vi "Receiver HMI Main.vi"() -> ()   [LabVIEW 2025]
uses:
  <vilib>/Instr/_visa.llb/VISA Configure Serial Port (Instr).vi
  <vilib>/picture/picture.llb/Draw True-Color Pixmap.vi
panel:
  out "Barcode":bool
  out "unsigned byte array":u8[](array[numeric])
  out "Wire":bool
  out "Motor":bool
  out "Light":bool
  out "Touch":bool
  out "Solenoid":bool
  out "Cancelled":bool
  out "Receive Buffer":string
  in  "Enable Wire":bool
  in  "Enable Barcode":bool
  in  "Enable Motor":bool
  in  "Enable Light":bool
  in  "Enable Touch":bool
  in  "Enable Solenoid":bool
  out "String":string
  out "2D Picture":picture
  out "Receiving Progress:":dbl(slide) scale=0.0..100.0
  # "RECEIVER"
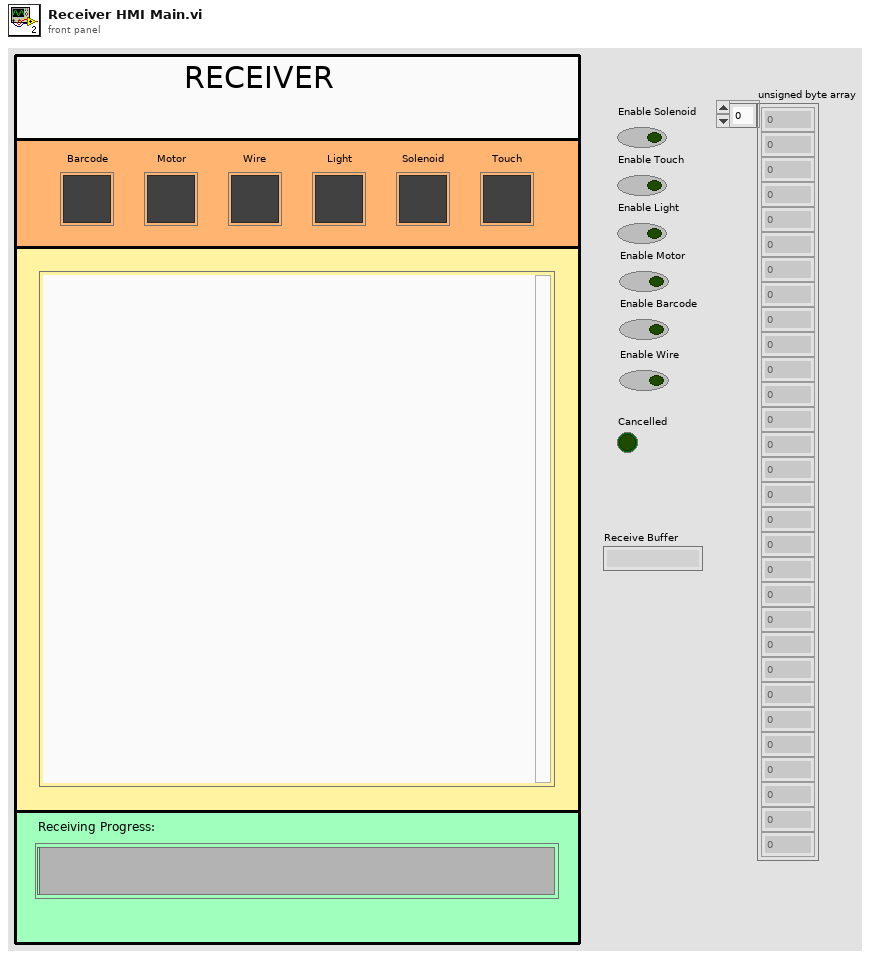
[diagram p1: front panel]
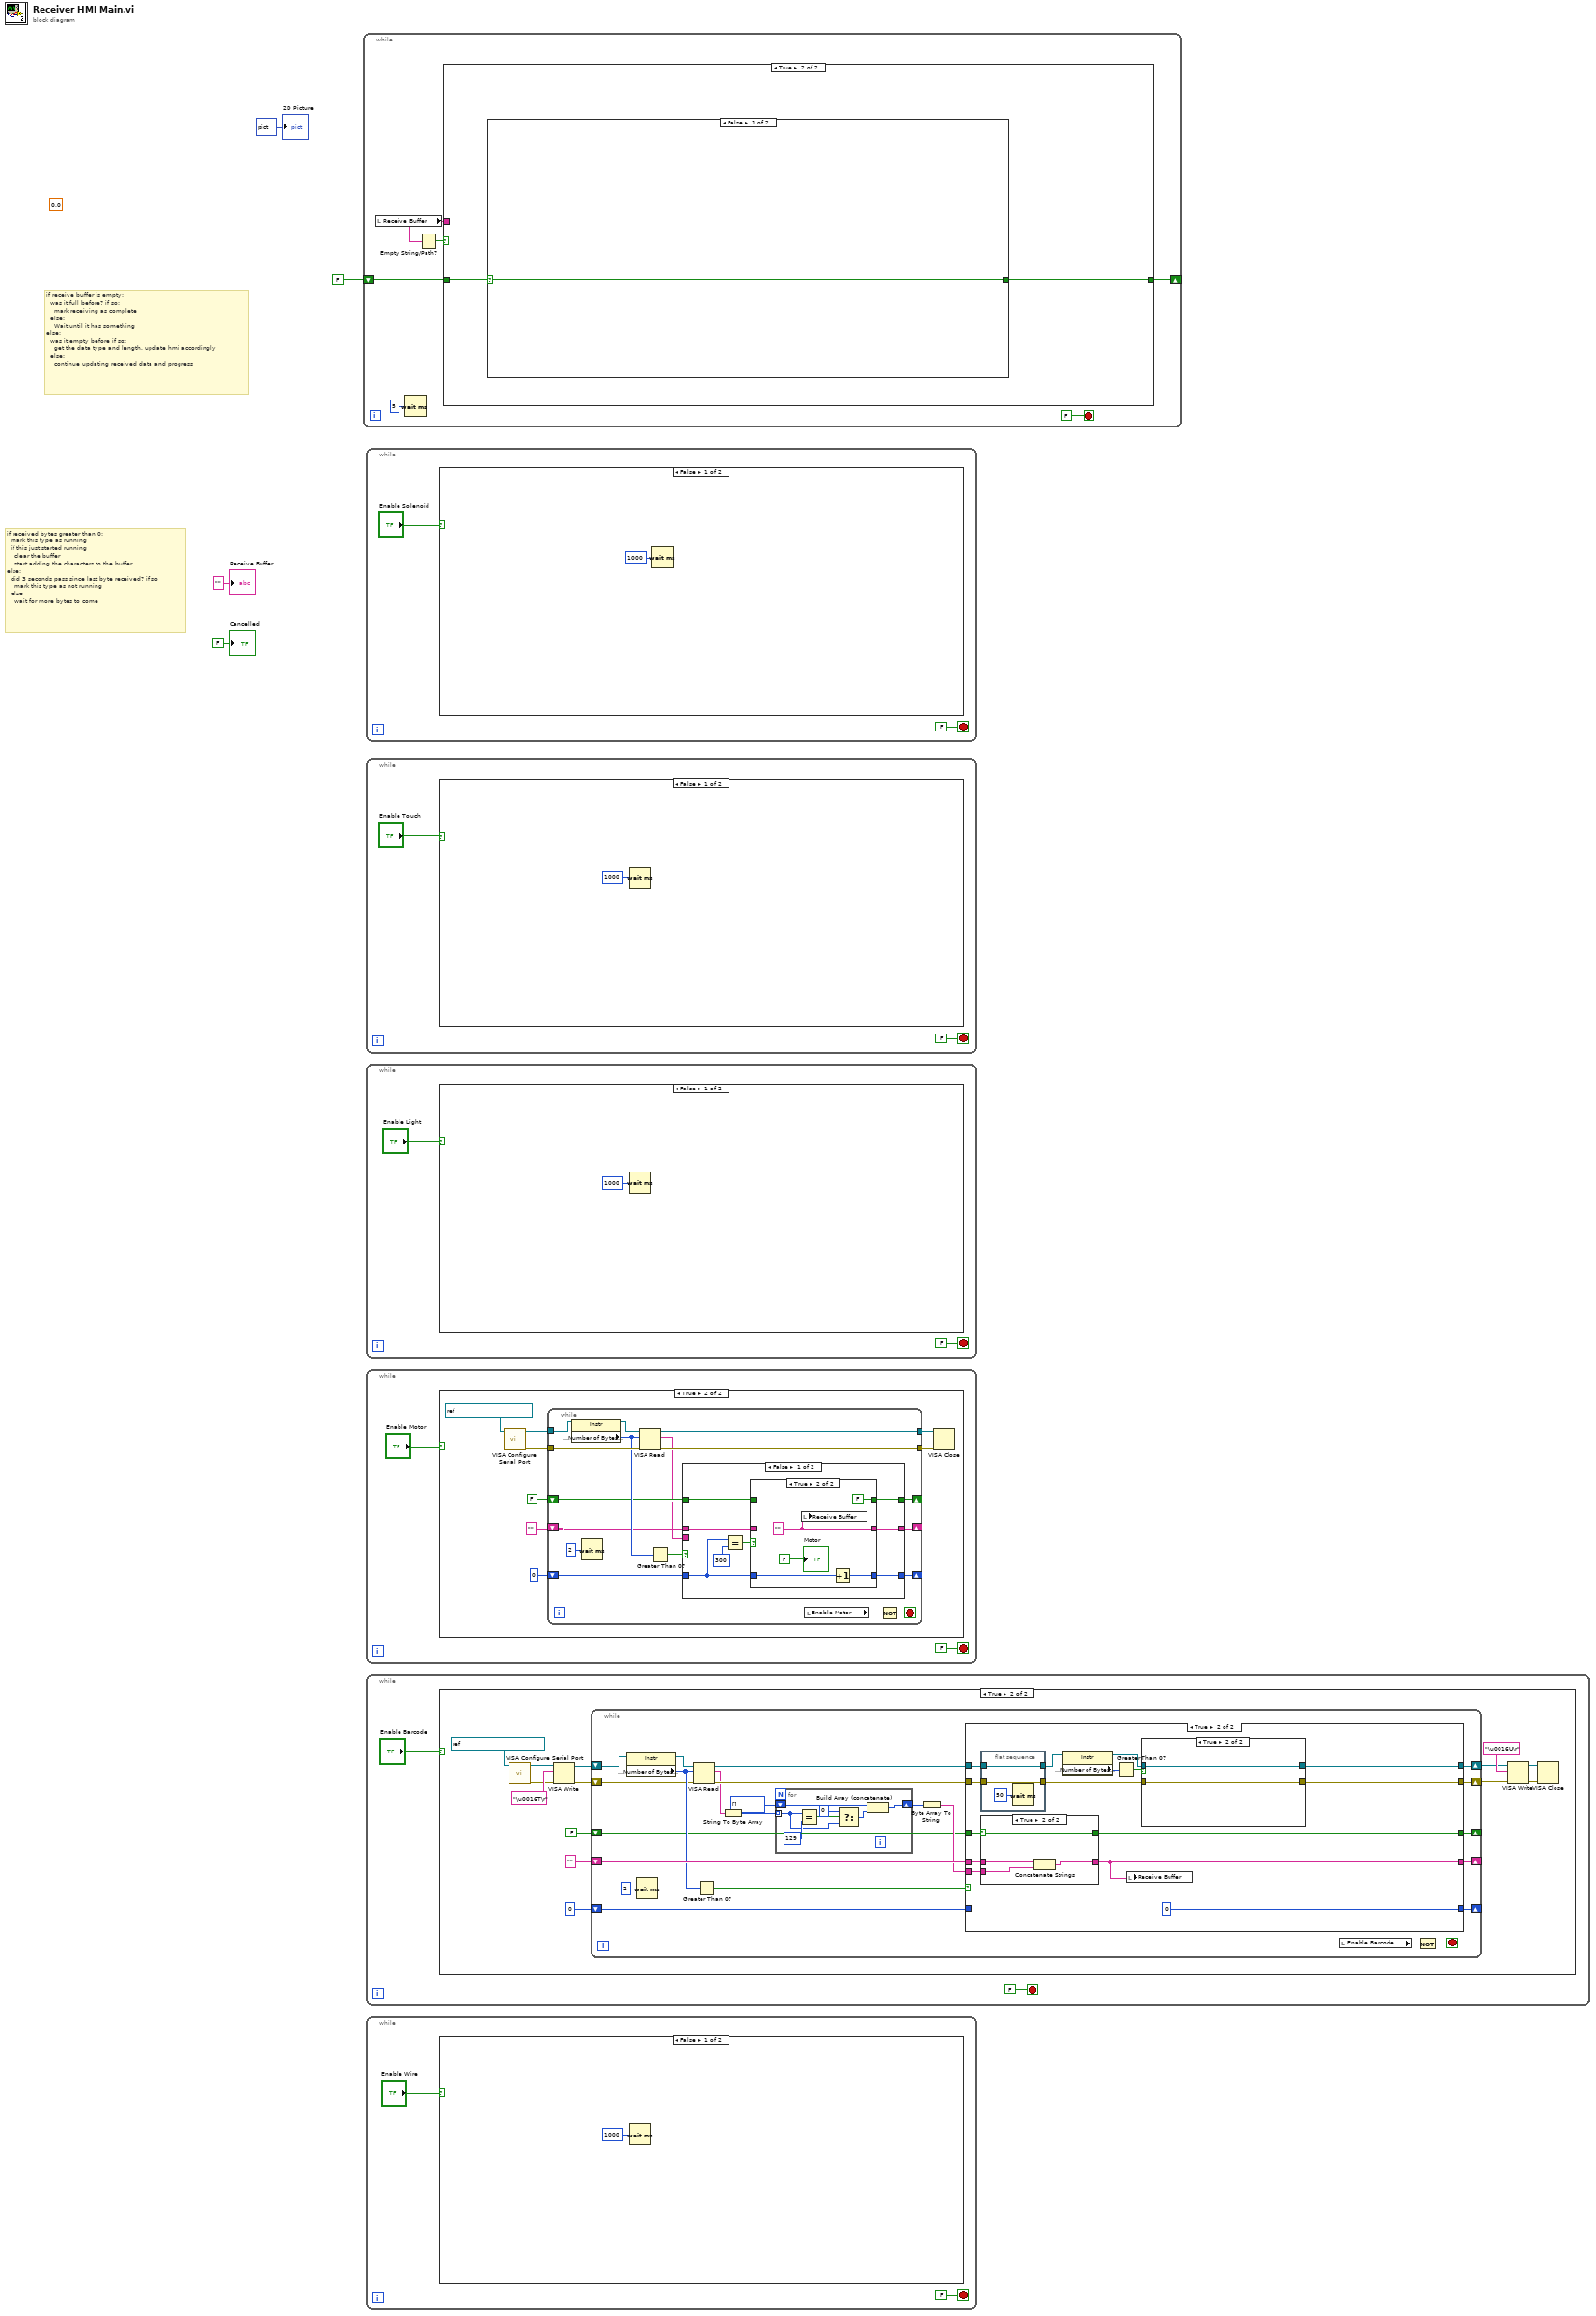
[diagram p0: block diagram]
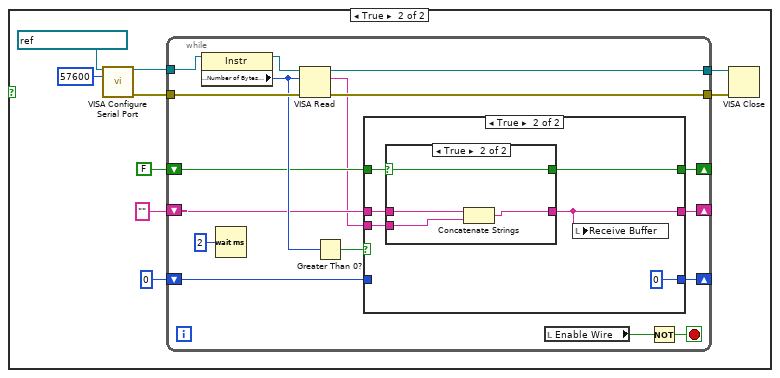
[diagram p2: hidden frame]
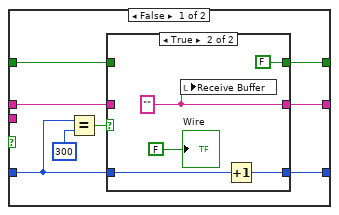
[diagram p3: hidden frame]
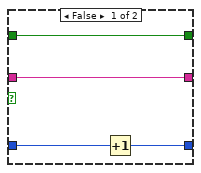
[diagram p4: hidden frame]
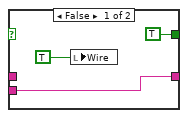
[diagram p5: hidden frame]
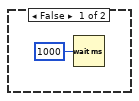
[diagram p6: hidden frame]
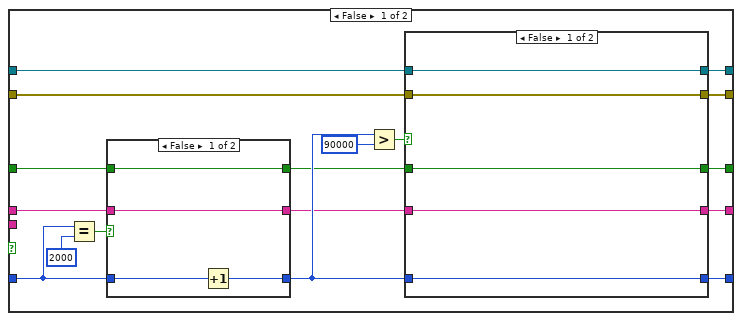
[diagram p7: hidden frame]
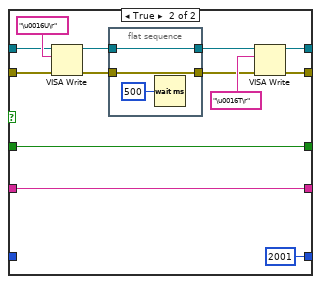
[diagram p8: hidden frame]
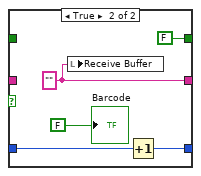
[diagram p9: hidden frame]
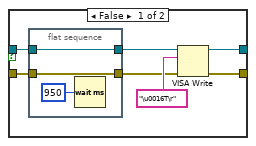
[diagram p10: hidden frame]
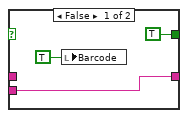
[diagram p11: hidden frame]
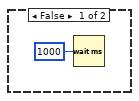
[diagram p12: hidden frame]
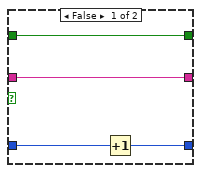
[diagram p13: hidden frame]
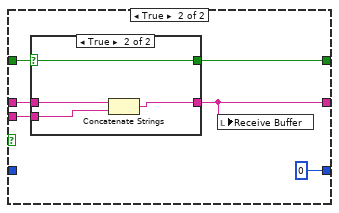
[diagram p14: hidden frame]
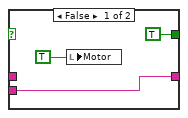
[diagram p15: hidden frame]
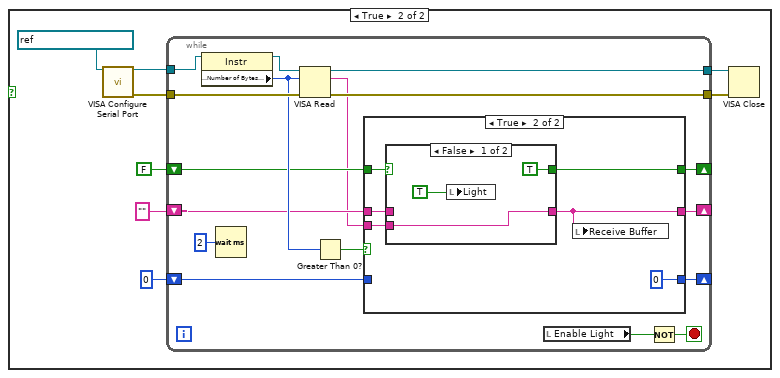
[diagram p16: hidden frame]
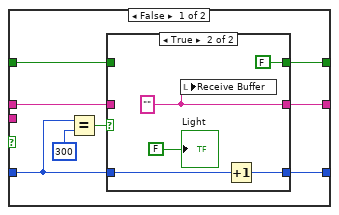
[diagram p17: hidden frame]
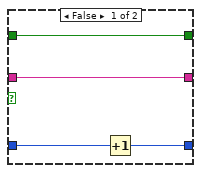
[diagram p18: hidden frame]
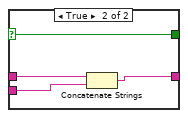
[diagram p19: hidden frame]
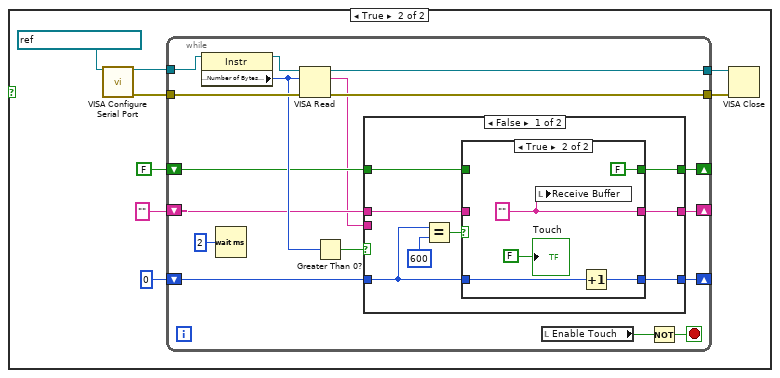
[diagram p20: hidden frame]
diagram:
  (unwired) 0.0 ("Receiving Progress:")
  # "if receive buffer is empty:\n  was it full before? if so:\n    mark receiving as complete\n  else:\n    Wait until it has something\nelse:\n  was it empty before if so:\n    get the data type and length. update hmi accordingly\n  else:\n    continue updating received data and progress"
  # "if received bytes greater than 0:\n  mark this type as running\n  if this just started running\n    clear the buffer\n    start adding the characters to the buffer\nelse:\n  did 3 seconds pass since last byte received? if so\n    mark this type as not running\n  else\n    wait for more bytes to come"
  n1 = while {
    shift-right: [w7] -> _
    shift-left: FALSE -> [w9]
    stop <- FALSE stop-if-true
    n2 = local read "Receive Buffer"() -> (w6:string)
    n3 = Wait (ms)(milliseconds to wait=u32 5) -> ()  [unwired: 1 out]
    n4 = Empty String/Path?(string/path=w6) -> (empty?=w10:bool)
    n5 = case shown="True" w10 {
      tunnel: w9 -> [_ w62]
      tunnel: [FALSE w61] -> w7
      tunnel: w6 -> [w12 _]
      frame False {
        n6 = String To Byte Array(string=w12) -> (unsigned byte array=→"unsigned byte array":u8[])
        n7 = String To Byte Array(string=w12) -> (unsigned byte array=w24:u8[])
        n8 = String Subset(string=w12, offset (0)=7) -> (substring=w18:string)  [unwired: 1 in]
        n9 = Index Array(array=w24, index=2) -> (element=w32:u8)
        n10 = Index Array(array=w24, index=3) -> (element=w20:u8)
        n11 = Index Array(array=w24, index=4) -> (element=w19:u8)
        n12 = Index Array(array=w24, index=5) -> (element=w26:u8)
        n13 = Index Array(array=w24, index=6) -> (element=w25:u8)
        n14 = Join Numbers(hi=w20, lo=w19) -> ((hi.lo)=w17:u16)
        n15 = Join Numbers(hi=w26, lo=w25) -> ((hi.lo)=w16:u16)
        n16 = String Length(string=w18) -> (length=w14:i32)
        n17 = case shown="0" w32 {
          tunnel: w24 -> [_ _ _]
          tunnel: w18 -> [w48 _ w58]
          tunnel: w17 -> [w34 _ w56]
          tunnel: w16 -> [w36 _ w55]
          tunnel: [w44 u32 0 w54] -> w15
          frame 1 {
            (unwired) FALSE
            n18 = To Long Integer(number=w34) -> (32bit integer=w35:i32)
            n19 = To Long Integer(number=w36) -> (32bit integer=w37:i32)
            n20 = Greater?(x=w34, y=w36) -> (0:w42:bool)
            n21 = call "Received String to 2D Pixmap Array.vi"("Width"=w34, "Height"=w36, "Receive Buffer"=w48) -> ("Array"=w47:u32[][])  [unwired: 8 in]
            n22 = Multiply(x=w35, y=w37) -> (x*y=w46:i32)
            n23 = Select(t=w34, s=w42, f=w36) -> (s? t:f=w38:u16)
            n24 = Multiply(x=u16 3, y=w46) -> (x*y=w44:i32)
            n25 = call-poly <vilib>:"Draw Unflattened Pixmap.vi"("data (RGB format)"=w47) -> ("new picture"=w49:picture)  [unwired: 8 in]
            n26 = Increment(x=w38) -> (x+1=w39:u16)
            n27 = Divide(x=u16 512, y=w39) -> (x/y=w40:dbl)
            n28 = local write "2D Picture"(w49) -> ()
            n29 = property on="2D Picture" class="Pict"("Visible"=TRUE) -> ()  [unwired: 2 in, 2 out]
            n30 = property on="2D Picture" class="Pict"("ZoomFactor"=w40) -> ()  [unwired: 2 in, 2 out]
            n31 = property on="String" class="Str"("Visible"=FALSE) -> ()  [unwired: 2 in, 2 out]
          }
          frame Default {
            (unwired) FALSE
            n32 = local write "String"("INVALID DATA TYPE") -> ()
          }
          frame 0 {
            (unwired) TRUE
            n33 = property on="2D Picture" class="Pict"("Visible"=FALSE) -> ()  [unwired: 2 in, 2 out]
            n34 = property on="String" class="Str"("Visible"=TRUE) -> ()  [unwired: 2 in, 2 out]
            n35 = Join Numbers(hi=w56, lo=w55) -> ((hi.lo)=w54:u32)
            n36 = property on="String" class="Str"() -> ("Key Focus"=w59:bool)  [unwired: 2 in, 2 out]
            n37 = case shown="False" w59 {
              frame False {
                n38 = property on="String" class="Str"("Text.Scroll Position"=u32 65535) -> ()  [unwired: 2 in, 2 out]
              }
              frame True {
              }
            }
            "String" <- w58
          }
        }
        n39 = Divide(x=w14, y=w15) -> (x/y=w31:dbl)
        n40 = Multiply(x=w31, y=100.0) -> (x*y=→"Receiving Progress:":dbl)
      }
      frame True {
        n41 = case shown="False" w62 {
          selector: w62 -> [w63 _]
          tunnel: [w63 FALSE] -> w61
          frame False {
          }
          frame True {
            # "mark receiving as complete"
          }
        }
      }
    }
  }
  n42 = while {
    stop <- FALSE stop-if-true
    n43 = case shown="False" "Enable Solenoid" {
      frame False {
        n44 = Wait (ms)(milliseconds to wait=u32 1000) -> ()  [unwired: 1 out]
      }
      frame True {
        n45 = call-poly "VISA Configure Serial Port"("VISA resource name"=refnum<visa-resource-name> "SOLENOID_RECEIVER") -> ("VISA resource name out"=w74:refnum<visa-resource-name>, "error out"=w75:errorcluster)  [unwired: 13 in]
        n46 = while {
          tunnel: w75 -> [w92]
          tunnel: w74 -> [w90]
          shift-right: [w79] -> _
          shift-left: 0 -> [w78]
          shift-right: [w82] -> _
          shift-left: "" -> [w83]
          tunnel: [w88] -> w71
          tunnel: [w87] -> w70
          shift-right: [w80] -> _
          shift-left: FALSE -> [w84]
          stop <- w77 stop-if-true
          n47 = property class="Instr"(reference=w90) -> (reference out=w89:refnum<visa-resource-name>, "Serial Settings:Number of Bytes at Serial Port"=w85:u32)  [unwired: 1 in, 1 out]
          n48 = Wait (ms)(milliseconds to wait=u32 2) -> ()  [unwired: 1 out]
          n49 = VISA Read(VISA resource name=w89, byte count=w85, error in (no error)=w92) -> (VISA resource name out=w88:refnum<visa-resource-name>, read buffer=w81:string, error out=w87:errorcluster)  [unwired: 1 out]
          n50 = Greater Than 0?(x=w85) -> (x > 0?=w86:bool)
          n51 = case shown="True" w86 {
            tunnel: w84 -> [w93 w115]
            tunnel: w83 -> [w98 w114]
            tunnel: [w97 w110] -> w82
            tunnel: w81 -> [_ w113]
            tunnel: [w96 w112] -> w80
            tunnel: [w95 0] -> w79
            tunnel: w78 -> [w94 _]
            frame False {
              n52 = Equal?(x=w94, y=300) -> (x = y?=w99:bool)
              n53 = case shown="False" w99 {
                tunnel: w98 -> [w104 _]
                tunnel: [w104 w107] -> w97
                tunnel: [w103 FALSE] -> w96
                tunnel: [w101 w105] -> w95
                tunnel: w94 -> [w102 w106]
                tunnel: w93 -> [w103 _]
                frame False {
                  n54 = Increment(x=w102) -> (x+1=w101:i32)
                }
                frame True {
                  w107 = ""
                  n55 = local write "Receive Buffer"(w107) -> ()
                  n56 = Increment(x=w106) -> (x+1=w105:i32)
                  "Solenoid" <- FALSE ("Solenoid")
                }
              }
            }
            frame True {
              n57 = case shown="False" w115 {
                selector: w115 -> [_ w122]
                tunnel: w114 -> [_ w121]
                tunnel: [w116 w120] -> w110
                tunnel: w113 -> [w116 w119]
                tunnel: [TRUE w122] -> w112
                frame False {
                  n58 = local write "Solenoid"(TRUE ("Solenoid")) -> ()
                }
                frame True {
                  n59 = Concatenate Strings(w121, w119) -> (w120:string)
                }
              }
              n60 = local write "Receive Buffer"(w110) -> ()
            }
          }
          n61 = local read "Enable Solenoid"() -> (w76:bool)
          n62 = Not(x=w76) -> (.not. x?=w77:bool)
        }
        n63 = VISA Close(VISA resource name=w71, error in (no error)=w70) -> ()  [unwired: 1 out]
      }
    }
  }
  n64 = while {
    stop <- FALSE stop-if-true
    n65 = case shown="False" "Enable Touch" {
      frame False {
        n66 = Wait (ms)(milliseconds to wait=u32 1000) -> ()  [unwired: 1 out]
      }
      frame True {
        n67 = call-poly "VISA Configure Serial Port"("VISA resource name"=refnum<visa-resource-name> "TOUCH_RECEIVER") -> ("VISA resource name out"=w132:refnum<visa-resource-name>, "error out"=w133:errorcluster)  [unwired: 13 in]
        n68 = while {
          tunnel: w133 -> [w150]
          tunnel: w132 -> [w148]
          shift-right: [w137] -> _
          shift-left: 0 -> [w136]
          shift-right: [w140] -> _
          shift-left: "" -> [w141]
          tunnel: [w146] -> w129
          tunnel: [w145] -> w128
          shift-right: [w138] -> _
          shift-left: FALSE -> [w142]
          stop <- w135 stop-if-true
          n69 = property class="Instr"(reference=w148) -> (reference out=w147:refnum<visa-resource-name>, "Serial Settings:Number of Bytes at Serial Port"=w143:u32)  [unwired: 1 in, 1 out]
          n70 = Wait (ms)(milliseconds to wait=u32 2) -> ()  [unwired: 1 out]
          n71 = VISA Read(VISA resource name=w147, byte count=w143, error in (no error)=w150) -> (VISA resource name out=w146:refnum<visa-resource-name>, read buffer=w139:string, error out=w145:errorcluster)  [unwired: 1 out]
          n72 = Greater Than 0?(x=w143) -> (x > 0?=w144:bool)
          n73 = case shown="False" w144 {
            tunnel: w142 -> [w154 w173]
            tunnel: w141 -> [w158 w172]
            tunnel: [w157 w168] -> w140
            tunnel: w139 -> [_ w171]
            tunnel: [w156 w170] -> w138
            tunnel: [w155 0] -> w137
            tunnel: w136 -> [w152 _]
            frame False {
              n74 = Equal?(x=w152, y=600) -> (x = y?=w153:bool)
              n75 = case shown="True" w153 {
                tunnel: w158 -> [w162 _]
                tunnel: [w162 w166] -> w157
                tunnel: [w161 FALSE] -> w156
                tunnel: [w159 w163] -> w155
                tunnel: w152 -> [w160 w164]
                tunnel: w154 -> [w161 _]
                frame False {
                  n76 = Increment(x=w160) -> (x+1=w159:i32)
                }
                frame True {
                  w166 = ""
                  n77 = local write "Receive Buffer"(w166) -> ()
                  n78 = Increment(x=w164) -> (x+1=w163:i32)
                  "Touch" <- FALSE ("Solenoid")
                }
              }
            }
            frame True {
              n79 = case shown="False" w173 {
                selector: w173 -> [_ w180]
                tunnel: w172 -> [_ w179]
                tunnel: [w174 w178] -> w168
                tunnel: w171 -> [w174 w177]
                tunnel: [TRUE w180] -> w170
                frame False {
                  n80 = local write "Touch"(TRUE ("Solenoid")) -> ()
                }
                frame True {
                  n81 = Concatenate Strings(w179, w177) -> (w178:string)
                }
              }
              n82 = local write "Receive Buffer"(w168) -> ()
            }
          }
          n83 = local read "Enable Touch"() -> (w134:bool)
          n84 = Not(x=w134) -> (.not. x?=w135:bool)
        }
        n85 = VISA Close(VISA resource name=w129, error in (no error)=w128) -> ()  [unwired: 1 out]
      }
    }
  }
  n86 = while {
    stop <- FALSE stop-if-true
    n87 = case shown="False" "Enable Light" {
      frame False {
        n88 = Wait (ms)(milliseconds to wait=u32 1000) -> ()  [unwired: 1 out]
      }
      frame True {
        n89 = call-poly "VISA Configure Serial Port"("VISA resource name"=refnum<visa-resource-name> "LIGHT_RECEIVER") -> ("VISA resource name out"=w190:refnum<visa-resource-name>, "error out"=w191:errorcluster)  [unwired: 13 in]
        n90 = while {
          tunnel: w191 -> [w208]
          tunnel: w190 -> [w206]
          shift-right: [w195] -> _
          shift-left: 0 -> [w194]
          shift-right: [w198] -> _
          shift-left: "" -> [w199]
          tunnel: [w204] -> w187
          tunnel: [w203] -> w186
          shift-right: [w196] -> _
          shift-left: FALSE -> [w200]
          stop <- w193 stop-if-true
          n91 = property class="Instr"(reference=w206) -> (reference out=w205:refnum<visa-resource-name>, "Serial Settings:Number of Bytes at Serial Port"=w201:u32)  [unwired: 1 in, 1 out]
          n92 = Wait (ms)(milliseconds to wait=u32 2) -> ()  [unwired: 1 out]
          n93 = VISA Read(VISA resource name=w205, byte count=w201, error in (no error)=w208) -> (VISA resource name out=w204:refnum<visa-resource-name>, read buffer=w197:string, error out=w203:errorcluster)  [unwired: 1 out]
          n94 = Greater Than 0?(x=w201) -> (x > 0?=w202:bool)
          n95 = case shown="True" w202 {
            tunnel: w200 -> [w212 w231]
            tunnel: w199 -> [w216 w230]
            tunnel: [w215 w226] -> w198
            tunnel: w197 -> [_ w229]
            tunnel: [w214 w228] -> w196
            tunnel: [w213 0] -> w195
            tunnel: w194 -> [w210 _]
            frame False {
              n96 = Equal?(x=w210, y=300) -> (x = y?=w211:bool)
              n97 = case shown="True" w211 {
                tunnel: w216 -> [w220 _]
                tunnel: [w220 w224] -> w215
                tunnel: [w219 FALSE] -> w214
                tunnel: [w217 w222] -> w213
                tunnel: w210 -> [w218 w223]
                tunnel: w212 -> [w219 _]
                frame False {
                  n98 = Increment(x=w218) -> (x+1=w217:i32)
                }
                frame True {
                  w224 = ""
                  n99 = local write "Receive Buffer"(w224) -> ()
                  n100 = Increment(x=w223) -> (x+1=w222:i32)
                  "Light" <- FALSE ("Solenoid")
                }
              }
            }
            frame True {
              n101 = case shown="False" w231 {
                selector: w231 -> [_ w238]
                tunnel: w230 -> [_ w237]
                tunnel: [w232 w236] -> w226
                tunnel: w229 -> [w232 w235]
                tunnel: [TRUE w238] -> w228
                frame False {
                  n102 = local write "Light"(TRUE ("Solenoid")) -> ()
                }
                frame True {
                  n103 = Concatenate Strings(w237, w235) -> (w236:string)
                }
              }
              n104 = local write "Receive Buffer"(w226) -> ()
            }
          }
          n105 = local read "Enable Light"() -> (w192:bool)
          n106 = Not(x=w192) -> (.not. x?=w193:bool)
        }
        n107 = VISA Close(VISA resource name=w187, error in (no error)=w186) -> ()  [unwired: 1 out]
      }
    }
  }
  n108 = while {
    stop <- FALSE stop-if-true
    n109 = case shown="True" "Enable Motor" {
      frame False {
        n110 = Wait (ms)(milliseconds to wait=u32 1000) -> ()  [unwired: 1 out]
      }
      frame True {
        n111 = call-poly "VISA Configure Serial Port"("VISA resource name"=refnum<visa-resource-name> "MOTOR_RECEIVER") -> ("VISA resource name out"=w248:refnum<visa-resource-name>, "error out"=w249:errorcluster)  [unwired: 13 in]
        n112 = while {
          tunnel: w249 -> [w266]
          tunnel: w248 -> [w264]
          shift-right: [w253] -> _
          shift-left: 0 -> [w252]
          shift-right: [w256] -> _
          shift-left: "" -> [w257]
          tunnel: [w262] -> w245
          tunnel: [w261] -> w244
          shift-right: [w254] -> _
          shift-left: FALSE -> [w258]
          stop <- w251 stop-if-true
          n113 = property class="Instr"(reference=w264) -> (reference out=w263:refnum<visa-resource-name>, "Serial Settings:Number of Bytes at Serial Port"=w259:u32)  [unwired: 1 in, 1 out]
          n114 = Wait (ms)(milliseconds to wait=u32 2) -> ()  [unwired: 1 out]
          n115 = VISA Read(VISA resource name=w263, byte count=w259, error in (no error)=w266) -> (VISA resource name out=w262:refnum<visa-resource-name>, read buffer=w255:string, error out=w261:errorcluster)  [unwired: 1 out]
          n116 = Greater Than 0?(x=w259) -> (x > 0?=w260:bool)
          n117 = case shown="False" w260 {
            tunnel: w258 -> [w270 w289]
            tunnel: w257 -> [w274 w288]
            tunnel: [w273 w284] -> w256
            tunnel: w255 -> [_ w287]
            tunnel: [w272 w286] -> w254
            tunnel: [w271 0] -> w253
            tunnel: w252 -> [w268 _]
            frame False {
              n118 = Equal?(x=w268, y=300) -> (x = y?=w269:bool)
              n119 = case shown="True" w269 {
                tunnel: w274 -> [w278 _]
                tunnel: [w278 w282] -> w273
                tunnel: [w277 FALSE] -> w272
                tunnel: [w275 w280] -> w271
                tunnel: w268 -> [w276 w281]
                tunnel: w270 -> [w277 _]
                frame False {
                  n120 = Increment(x=w276) -> (x+1=w275:i32)
                }
                frame True {
                  w282 = ""
                  n121 = local write "Receive Buffer"(w282) -> ()
                  n122 = Increment(x=w281) -> (x+1=w280:i32)
                  "Motor" <- FALSE ("Solenoid")
                }
              }
            }
            frame True {
              n123 = case shown="True" w289 {
                selector: w289 -> [_ w296]
                tunnel: w288 -> [_ w295]
                tunnel: [w290 w294] -> w284
                tunnel: w287 -> [w290 w293]
                tunnel: [TRUE w296] -> w286
                frame False {
                  n124 = local write "Motor"(TRUE ("Solenoid")) -> ()
                }
                frame True {
                  n125 = Concatenate Strings(w295, w293) -> (w294:string)
                }
              }
              n126 = local write "Receive Buffer"(w284) -> ()
            }
          }
          n127 = local read "Enable Motor"() -> (w250:bool)
          n128 = Not(x=w250) -> (.not. x?=w251:bool)
        }
        n129 = VISA Close(VISA resource name=w245, error in (no error)=w244) -> ()  [unwired: 1 out]
      }
    }
  }
  n130 = while {
    stop <- FALSE stop-if-true
    n131 = case shown="True" "Enable Barcode" {
      frame False {
        n132 = Wait (ms)(milliseconds to wait=u32 1000) -> ()  [unwired: 1 out]
      }
      frame True {
        n133 = call-poly "VISA Configure Serial Port"("VISA resource name"=refnum<visa-resource-name> "BARCODE_RECEIVER") -> ("VISA resource name out"=w307:refnum<visa-resource-name>, "error out"=w309:errorcluster)  [unwired: 13 in]
        n134 = VISA Write(VISA resource name=w307, write buffer="\u0016T\r", error in (no error)=w309) -> (VISA resource name out=w306:refnum<visa-resource-name>, error out=w308:errorcluster)  [unwired: 1 out]
        n135 = while {
          shift-right: [w326] -> w304
          shift-left: w308 -> [w323]
          shift-right: [w325] -> w301
          shift-left: w306 -> [w322]
          shift-right: [w333] -> _
          shift-left: 0 -> [w335]
          shift-right: [w332] -> _
          shift-left: "" -> [w334]
          shift-right: [w315] -> _
          shift-left: FALSE -> [w314]
          stop <- w331 stop-if-true
          n136 = property class="Instr"(reference=w322) -> (reference out=w336:refnum<visa-resource-name>, "Serial Settings:Number of Bytes at Serial Port"=w328:u32)  [unwired: 1 in, 1 out]
          n137 = Wait (ms)(milliseconds to wait=u32 2) -> ()  [unwired: 1 out]
          n138 = VISA Read(VISA resource name=w336, byte count=w328, error in (no error)=w323) -> (VISA resource name out=w324:refnum<visa-resource-name>, read buffer=w320:string, error out=w327:errorcluster)  [unwired: 1 out]
          n139 = Greater Than 0?(x=w328) -> (x > 0?=w329:bool)
          n140 = String To Byte Array(string=w320) -> (unsigned byte array=w319:u8[])
          n141 = for {
            tunnel: w319 -> [w340] mode=indexing
            shift-right: [w339] -> w317
            shift-left: u8[] [] ("unsigned byte array") -> [w338]
            n142 = Equal?(x=w340, y=u8 129) -> (x = y?=w342:bool)
            n143 = Select(t=u8 0, s=w342, f=w340) -> (s? t:f=w337:u8)
            n144 = Build Array (concatenate)(w338, w337) -> (w339:u8[])
          }
          n145 = Byte Array To String(unsigned byte array=w317) -> (string=w316:string)
          n146 = case shown="True" w329 {
            tunnel: w314 -> [w359 w405]
            tunnel: w334 -> [w360 w404]
            tunnel: [w347 w400] -> w332
            tunnel: w316 -> [_ w403]
            tunnel: [w345 w402] -> w315
            tunnel: [w349 0] -> w333
            tunnel: w335 -> [w357 _]
            tunnel: w327 -> [w351 w397]
            tunnel: [w353 w399] -> w326
            tunnel: [w352 w398] -> w325
            tunnel: w324 -> [w350 w395]
            frame False {
              n147 = Equal?(x=w357, y=2000) -> (x = y?=w358:bool)
              n148 = case shown="False" w358 {
                tunnel: w360 -> [w385 _]
                tunnel: [w385 w386] -> w346
                tunnel: [w384 FALSE] -> w344
                tunnel: [w382 w388] -> w348
                tunnel: w357 -> [w383 w389]
                tunnel: w359 -> [w384 _]
                frame False {
                  n149 = Increment(x=w383) -> (x+1=w382:i32)
                }
                frame True {
                  w386 = ""
                  n150 = local write "Receive Buffer"(w386) -> ()
                  n151 = Increment(x=w389) -> (x+1=w388:i32)
                  "Barcode" <- FALSE ("Solenoid")
                }
              }
              n152 = Greater?(x=w348, y=90000) -> (0:w354:bool)
              n153 = case shown="False" w354 {
                tunnel: [w365 w376] -> w353
                tunnel: [w364 w375] -> w352
                tunnel: w351 -> [w365 w370]
                tunnel: w350 -> [w364 w369]
                tunnel: [w361 2001] -> w349
                tunnel: w348 -> [w361 _]
                tunnel: [w362 w368] -> w347
                tunnel: w346 -> [w362 w368]
                tunnel: [w363 w367] -> w345
                tunnel: w344 -> [w363 w367]
                frame False {
                }
                frame True {
                  n154 = VISA Write(VISA resource name=w369, write buffer="\u0016U\r", error in (no error)=w370) -> (VISA resource name out=w371:refnum<visa-resource-name>, error out=w373:errorcluster)  [unwired: 1 out]
                  n155 = flat-sequence {
                    tunnel: w373 -> [w381]
                    tunnel: [w381] -> w374
                    tunnel: w371 -> [w379]
                    tunnel: [w379] -> w372
                    frame #0 {
                      n156 = Wait (ms)(milliseconds to wait=u32 500) -> ()  [unwired: 1 out]
                    }
                  }
                  n157 = VISA Write(VISA resource name=w372, write buffer="\u0016T\r", error in (no error)=w374) -> (VISA resource name out=w375:refnum<visa-resource-name>, error out=w376:errorcluster)  [unwired: 1 out]
                }
              }
            }
            frame True {
              n158 = case shown="True" w405 {
                selector: w405 -> [_ w427]
                tunnel: w404 -> [_ w426]
                tunnel: [w421 w425] -> w400
                tunnel: w403 -> [w421 w424]
                tunnel: [TRUE w427] -> w402
                frame False {
                  n159 = local write "Barcode"(TRUE ("Solenoid")) -> ()
                }
                frame True {
                  n160 = Concatenate Strings(w426, w424) -> (w425:string)
                }
              }
              n161 = flat-sequence {
                tunnel: w397 -> [w420]
                tunnel: [w420] -> w396
                tunnel: w395 -> [w418]
                tunnel: [w418] -> w394
                frame #0 {
                  n162 = Wait (ms)(milliseconds to wait=u32 50) -> ()  [unwired: 1 out]
                }
              }
              n163 = property class="Instr"(reference=w394) -> (reference out=w391:refnum<visa-resource-name>, "Serial Settings:Number of Bytes at Serial Port"=w393:u32)  [unwired: 1 in, 1 out]
              n164 = Greater Than 0?(x=w393) -> (x > 0?=w392:bool)
              n165 = local write "Receive Buffer"(w400) -> ()
              n166 = case shown="True" w392 {
                tunnel: [w412 w417] -> w399
                tunnel: [w411 w416] -> w398
                tunnel: w396 -> [w409 w417]
                tunnel: w391 -> [w406 w416]
                frame False {
                  n167 = flat-sequence {
                    tunnel: w409 -> [w415]
                    tunnel: [w415] -> w408
                    tunnel: w406 -> [w413]
                    tunnel: [w413] -> w407
                    frame #0 {
                      n168 = Wait (ms)(milliseconds to wait=u32 950) -> ()  [unwired: 1 out]
                    }
                  }
                  n169 = VISA Write(VISA resource name=w407, write buffer="\u0016T\r", error in (no error)=w408) -> (VISA resource name out=w411:refnum<visa-resource-name>, error out=w412:errorcluster)  [unwired: 1 out]
                }
                frame True {
                }
              }
            }
          }
          n170 = local read "Enable Barcode"() -> (w330:bool)
          n171 = Not(x=w330) -> (.not. x?=w331:bool)
        }
        n172 = VISA Write(VISA resource name=w301, write buffer="\u0016U\r", error in (no error)=w304) -> (VISA resource name out=w302:refnum<visa-resource-name>, error out=w303:errorcluster)  [unwired: 1 out]
        n173 = VISA Close(VISA resource name=w302, error in (no error)=w303) -> ()  [unwired: 1 out]
      }
    }
  }
  n174 = while {
    stop <- FALSE stop-if-true
    n175 = case shown="False" "Enable Wire" {
      frame False {
        n176 = Wait (ms)(milliseconds to wait=u32 1000) -> ()  [unwired: 1 out]
      }
      frame True {
        n177 = call-poly "VISA Configure Serial Port"("VISA resource name"=refnum<visa-resource-name> "WIRE_RECEIVER", "baud rate (9600)"=u32 57600) -> ("VISA resource name out"=w438:refnum<visa-resource-name>, "error out"=w439:errorcluster)  [unwired: 12 in]
        n178 = while {
          tunnel: w439 -> [w456]
          tunnel: w438 -> [w454]
          shift-right: [w443] -> _
          shift-left: 0 -> [w442]
          shift-right: [w446] -> _
          shift-left: "" -> [w447]
          tunnel: [w452] -> w435
          tunnel: [w451] -> w434
          shift-right: [w444] -> _
          shift-left: FALSE -> [w448]
          stop <- w441 stop-if-true
          n179 = property class="Instr"(reference=w454) -> (reference out=w453:refnum<visa-resource-name>, "Serial Settings:Number of Bytes at Serial Port"=w449:u32)  [unwired: 1 in, 1 out]
          n180 = Wait (ms)(milliseconds to wait=u32 2) -> ()  [unwired: 1 out]
          n181 = VISA Read(VISA resource name=w453, byte count=w449, error in (no error)=w456) -> (VISA resource name out=w452:refnum<visa-resource-name>, read buffer=w445:string, error out=w451:errorcluster)  [unwired: 1 out]
          n182 = Greater Than 0?(x=w449) -> (x > 0?=w450:bool)
          n183 = case shown="True" w450 {
            tunnel: w448 -> [w460 w479]
            tunnel: w447 -> [w464 w478]
            tunnel: [w463 w474] -> w446
            tunnel: w445 -> [_ w477]
            tunnel: [w462 w476] -> w444
            tunnel: [w461 0] -> w443
            tunnel: w442 -> [w458 _]
            frame False {
              n184 = Equal?(x=w458, y=300) -> (x = y?=w459:bool)
              n185 = case shown="True" w459 {
                tunnel: w464 -> [w468 _]
                tunnel: [w468 w472] -> w463
                tunnel: [w467 FALSE] -> w462
                tunnel: [w465 w470] -> w461
                tunnel: w458 -> [w466 w471]
                tunnel: w460 -> [w467 _]
                frame False {
                  n186 = Increment(x=w466) -> (x+1=w465:i32)
                }
                frame True {
                  w472 = ""
                  n187 = local write "Receive Buffer"(w472) -> ()
                  n188 = Increment(x=w471) -> (x+1=w470:i32)
                  "Wire" <- FALSE ("Solenoid")
                }
              }
            }
            frame True {
              n189 = case shown="True" w479 {
                selector: w479 -> [_ w486]
                tunnel: w478 -> [_ w485]
                tunnel: [w480 w484] -> w474
                tunnel: w477 -> [w480 w483]
                tunnel: [TRUE w486] -> w476
                frame False {
                  n190 = local write "Wire"(TRUE ("Solenoid")) -> ()
                }
                frame True {
                  n191 = Concatenate Strings(w485, w483) -> (w484:string)
                }
              }
              n192 = local write "Receive Buffer"(w474) -> ()
            }
          }
          n193 = local read "Enable Wire"() -> (w440:bool)
          n194 = Not(x=w440) -> (.not. x?=w441:bool)
        }
        n195 = VISA Close(VISA resource name=w435, error in (no error)=w434) -> ()  [unwired: 1 out]
      }
    }
  }
  "Cancelled" <- FALSE ("Cancelled")
  "Receive Buffer" <- "" ("read buffer")
  "2D Picture" <- picture data[5B] ("2D Picture")
